vi "Plant Catalog W3.vi"() -> ()   [LabVIEW 2021, in "Tree Map.lvlib"]
doc: "<b>Author:</b> Piotr Kruczkowski <PrimaryKey>\n<b>License:</b> NewBSD\n\nCopyright (c) 2019, National Instruments\nAll rights reserved.\n\nRedistribution and use in source and binary forms, with or without\nmodification, are permitted provided that the following conditions are met:\n1. Redistributions of source code must retain the above copyright\n notice, this list of conditions and the following disclaimer.\n2. Redistributions in binary form must reproduce the above copyright\n notice, this list of conditions and the following disclaimer in the\n documentation and/or other materials provided with the distribution.\n3. Neither the name of National Instruments nor the\n names of its contributors may be used to endorse or promote products\n derived from this software without specific prior written permission.\n\nTHIS SOFTWARE IS PROVIDED BY National Instruments ''AS IS'' AND ANY\nEXPRESS OR IMPLIED WARRANTIES, INCLUDING, BUT NOT LIMITED TO, THE IMPLIED\nWARRANTIES OF MERCHANTABILITY AND FITNESS FOR A PARTICULAR PURPOSE ARE\nDISCLAIMED. IN NO EVENT SHALL National Instruments BE LIABLE FOR ANY\nDIRECT, INDIRECT, INCIDENTAL, SPECIAL, EXEMPLARY, OR CONSEQUENTIAL DAMAGES\n(INCLUDING, BUT NOT LIMITED TO, PROCUREMENT OF SUBSTITUTE GOODS OR SERVICES;\nLOSS OF USE, DATA, OR PROFITS; OR BUSINESS INTERRUPTION) HOWEVER CAUSED AND\nON ANY THEORY OF LIABILITY, WHETHER IN CONTRACT, STRICT LIABILITY, OR TORT\n(INCLUDING NEGLIGENCE OR OTHERWISE) ARISING IN ANY WAY OUT OF THE USE OF THIS\nSOFTWARE, EVEN IF ADVISED OF THE POSSIBILITY OF SUCH DAMAGE."
uses:
  <vilib>/National Instruments/Tree Map/Tree Map.lvlib
  <vilib>/National Instruments/Tree Map/API/List Roots.vi
  <vilib>/National Instruments/Tree Map/Utility/Into Tree Control Items.vi
panel:
  out "Array":string[](array[string])
  out "COMMON Unique Paths Set":set{string}(c389)={"\\CATALOG\\PLANT\\COMMON", "\\CATALOG\\PLANT_000000\\COMMON", "\\CATALOG\\PLANT_000001\\COMMON", "\\CATALOG\\PLANT_000002\\COMMON", "\\CATALOG\\PLANT_000003\\COMMON", "\\CATALOG\\PLANT_000004\\COMMON", "\\CATALOG\\PLANT_000005\\COMMON", "\\CATALOG\\PLANT_000006\\COMMON", "\\CATALOG\\PLANT_000007\\COMMON", "\\CATALOG\\PLANT_000008\\COMMON", "\\CATALOG\\PLANT_000009\\COMMON", "\\CATALOG\\PLANT_000010\\COMMON", "\\CATALOG\\PLANT_000011\\COMMON", "\\CATALOG\\PLANT_000012\\COMMON", "\\CATALOG\\PLANT_000013\\COMMON", "\\CATALOG\\PLANT_000014\\COMMON", "\\CATALOG\\PLANT_000015\\COMMON", "\\CATALOG\\PLANT_000016\\COMMON", "\\CATALOG\\PLANT_000017\\COMMON", "\\CATALOG\\PLANT_000018\\COMMON", "\\CATALOG\\PLANT_000019\\COMMON", "\\CATALOG\\PLANT_000020\\COMMON", "\\CATALOG\\PLANT_000021\\COMMON", "\\CATALOG\\PLANT_000022\\COMMON", "\\CATALOG\\PLANT_000023\\COMMON", "\\CATALOG\\PLANT_000024\\COMMON", "\\CATALOG\\PLANT_000025\\COMMON", "\\CATALOG\\PLANT_000026\\COMMON", "\\CATALOG\\PLANT_000027\\COMMON", "\\CATALOG\\PLANT_000028\\COMMON", "\\CATALOG\\PLANT_000029\\COMMON", "\\CATALOG\\PLANT_000030\\COMMON", "\\CATALOG\\PLANT_000031\\COMMON", "\\CATALOG\\PLANT_000032\\COMMON", "\\CATALOG\\PLANT_000033\\COMMON", "\\CATALOG\\PLANT_000034\\COMMON"}
  out "Botanical Data":string[](array[string])=["Sanguinaria canadensis", "Aquilegia canadensis", "Caltha palustris", "Caltha palustris", "Dicentra cucullaria", "Asarum canadense", "Hepatica americana", "Hepatica americana", "Arisaema triphyllum", "Podophyllum peltatum", "Phlox divaricata", "Phlox divaricata", "Claytonia Virginica", "Trillium grandiflorum", "Trillium grandiflorum", "Erythronium americanum", "Erythronium americanum", "Erythronium americanum", "Anemone blanda", "Anemone blanda", "Monarda didyma", "Monarda didyma", "Rudbeckia hirta", "Ranunculus", "Ranunculus", "Asclepias tuberosa", "Potentilla", "Oenothera", "Gentiana", "Gentiana", "Polemonium caeruleum", "Polemonium caeruleum", "Eschscholzia californica", "Dodecatheon", "Cimicifuga", "Lobelia cardinalis"]
  out "BOTANICAL Unique Paths Set":set{string}(c389)={"\\CATALOG\\PLANT\\BOTANICAL", "\\CATALOG\\PLANT_000000\\BOTANICAL", "\\CATALOG\\PLANT_000001\\BOTANICAL", "\\CATALOG\\PLANT_000002\\BOTANICAL", "\\CATALOG\\PLANT_000003\\BOTANICAL", "\\CATALOG\\PLANT_000004\\BOTANICAL", "\\CATALOG\\PLANT_000005\\BOTANICAL", "\\CATALOG\\PLANT_000006\\BOTANICAL", "\\CATALOG\\PLANT_000007\\BOTANICAL", "\\CATALOG\\PLANT_000008\\BOTANICAL", "\\CATALOG\\PLANT_000009\\BOTANICAL", "\\CATALOG\\PLANT_000010\\BOTANICAL", "\\CATALOG\\PLANT_000011\\BOTANICAL", "\\CATALOG\\PLANT_000012\\BOTANICAL", "\\CATALOG\\PLANT_000013\\BOTANICAL", "\\CATALOG\\PLANT_000014\\BOTANICAL", "\\CATALOG\\PLANT_000015\\BOTANICAL", "\\CATALOG\\PLANT_000016\\BOTANICAL", "\\CATALOG\\PLANT_000017\\BOTANICAL", "\\CATALOG\\PLANT_000018\\BOTANICAL", "\\CATALOG\\PLANT_000019\\BOTANICAL", "\\CATALOG\\PLANT_000020\\BOTANICAL", "\\CATALOG\\PLANT_000021\\BOTANICAL", "\\CATALOG\\PLANT_000022\\BOTANICAL", "\\CATALOG\\PLANT_000023\\BOTANICAL", "\\CATALOG\\PLANT_000024\\BOTANICAL", "\\CATALOG\\PLANT_000025\\BOTANICAL", "\\CATALOG\\PLANT_000026\\BOTANICAL", "\\CATALOG\\PLANT_000027\\BOTANICAL", "\\CATALOG\\PLANT_000028\\BOTANICAL", "\\CATALOG\\PLANT_000029\\BOTANICAL", "\\CATALOG\\PLANT_000030\\BOTANICAL", "\\CATALOG\\PLANT_000031\\BOTANICAL", "\\CATALOG\\PLANT_000032\\BOTANICAL", "\\CATALOG\\PLANT_000033\\BOTANICAL", "\\CATALOG\\PLANT_000034\\BOTANICAL"}
  in  "Tree Control":string(tree)
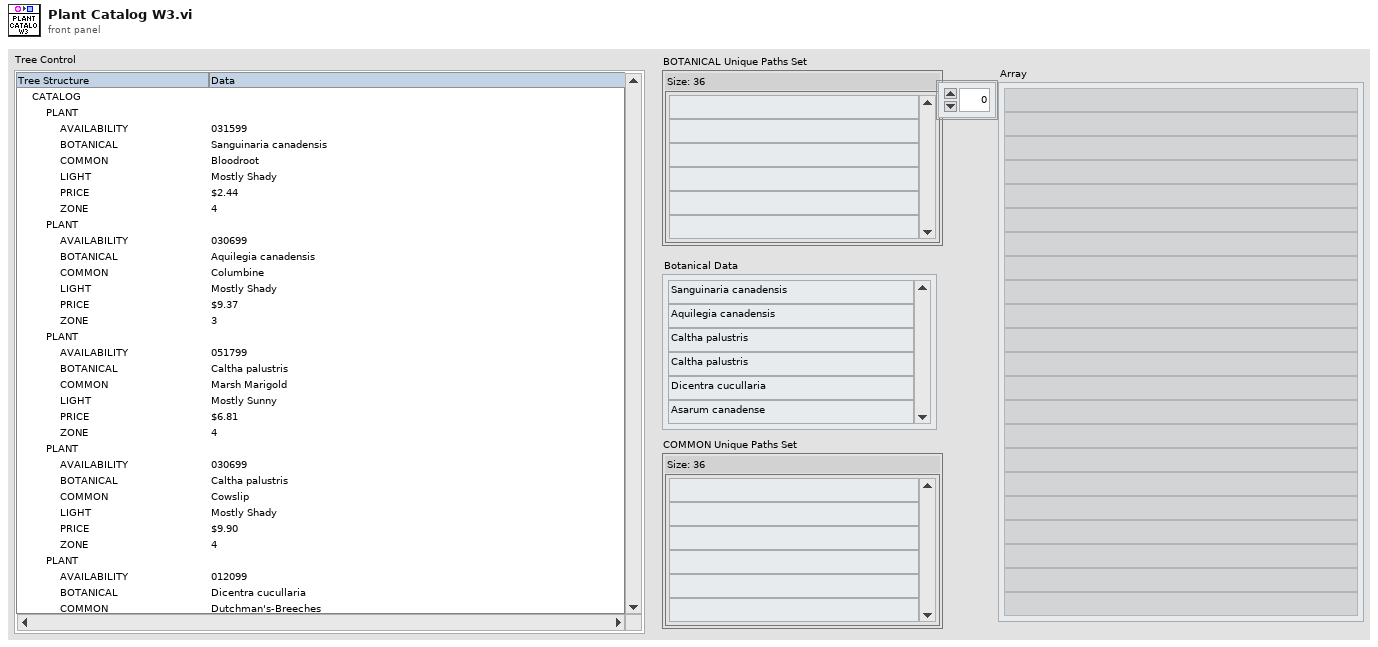
[diagram p1: front panel]
types:
  T1 = typedef "Tree Map.lvlib/Tree Map Data.ctl" = map{string, cluster{"Child Paths Set":set{string}, "Name":string, "Data":string, "Attributes":map{string, string}}}
  T2 = cluster{"Left Cell String":string, "Child Text":string[], "Child Tag":string, "Item Indent":i32, "Child Only?":bool, "Glyph Index":i32}[]
  T3 = cluster{"Child Paths Set":set{string}, "Name":string, "Data":string, "Attributes":map{string, string}}
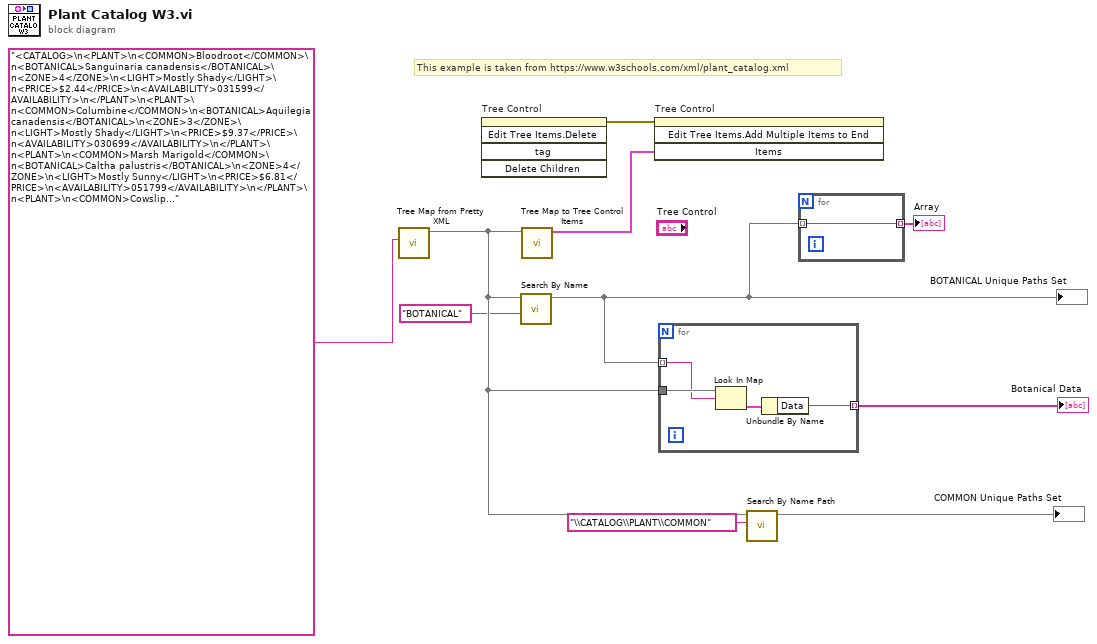
[diagram p0: block diagram]
diagram:
  # "This example is taken from https://www.w3schools.com/xml/plant_catalog.xml"
  n1 = call <vilib>:"Tree Map from Pretty XML.vi"("Pretty XML"="<CATALOG>\n<PLANT>\n<COMMON>Bloodroot</COMMON>\n<BOTANICAL>Sanguinaria canadensis</BOTANICAL>\n<ZONE>4</ZONE>\n<LIGHT>Mostly Shady</LIGHT>\n<PRICE>$2.44</PRICE>\n<AVAILABILITY>031599</AVAILABILITY>\n</PLANT>\n<PLANT>\n<COMMON>Columbine</COMMON>\n<BOTANICAL>Aquilegia canadensis</BOTANICAL>\n<ZONE>3</ZONE>\n<LIGHT>Mostly Shady</LIGHT>\n<PRICE>$9.37</PRICE>\n<AVAILABILITY>030699</AVAILABILITY>\n</PLANT>\n<PLANT>\n<COMMON>Marsh Marigold</COMMON>\n<BOTANICAL>Caltha palustris</BOTANICAL>\n<ZONE>4</ZONE>\n<LIGHT>Mostly Sunny</LIGHT>\n<PRICE>$6.81</PRICE>\n<AVAILABILITY>051799</AVAILABILITY>\n</PLANT>\n<PLANT>\n<COMMON>Cowslip</COMMON>\n<BOTANICAL>Caltha palustris</BOTANICAL>\n<ZONE>4</ZONE>\n<LIGHT>Mostly Shady</LIGHT>\n<PRICE>$9.90</PRICE>\n<AVAILABILITY>030699</AVAILABILITY>\n</PLANT>\n<PLANT>\n<COMMON>Dutchman's-Breeches</COMMON>\n<BOTANICAL>Dicentra cucullaria</BOTANICAL>\n<ZONE>3</ZONE>\n<LIGHT>Mostly Shady</LIGHT>\n<PRICE>$6.44</PRICE>\n<AVAILABILITY>012099</AVAILABILITY>\n</PLANT>\n<PLANT>\n<COMMON>Ginger, Wild</COMMON>\n<BOTANICAL>Asarum canadense</BOTANICAL>\n<ZONE>3</ZONE>\n<LIGHT>Mostly Shady</LIGHT>\n<PRICE>$9.03</PRICE>\n<AVAILABILITY>041899</AVAILABILITY>\n</PLANT>\n<PLANT>\n<COMMON>Hepatica</COMMON>\n<BOTANICAL>Hepatica americana</BOTANICAL>\n<ZONE>4</ZONE>\n<LIGHT>Mostly Shady</LIGHT>\n<PRICE>$4.45</PRICE>\n<AVAILABILITY>012699</AVAILABILITY>\n</PLANT>\n<PLANT>\n<COMMON>Liverleaf</COMMON>\n<BOTANICAL>Hepatica americana</BOTANICAL>\n<ZONE>4</ZONE>\n<LIGHT>Mostly Shady</LIGHT>\n<PRICE>$3.99</PRICE>\n<AVAILABILITY>010299</AVAILABILITY>\n</PLANT>\n<PLANT>\n<COMMON>Jack-In-The-Pulpit</COMMON>\n<BOTANICAL>Arisaema triphyllum</BOTANICAL>\n<ZONE>4</ZONE>\n<LIGHT>Mostly Shady</LIGHT>\n<PRICE>$3.23</PRICE>\n<AVAILABILITY>020199</AVAILABILITY>\n</PLANT>\n<PLANT>\n<COMMON>Mayapple</COMMON>\n<BOTANICAL>Podophyllum peltatum</BOTANICAL>\n<ZONE>3</ZONE>\n<LIGHT>Mostly Shady</LIGHT>\n<PRICE>$2.98</PRICE>\n<AVAILABILITY>060599</AVAILABILITY>\n</PLANT>\n<PLANT>\n<COMMON>Phlox, Woodland</COMMON>\n<BOTANICAL>Phlox divaricata</BOTANICAL>\n<ZONE>3</ZONE>\n<LIGHT>Sun or Shade</LIGHT>\n<PRICE>$2.80</PRICE>\n<AVAILABILITY>012299</AVAILABILITY>\n</PLANT>\n<PLANT>\n<COMMON>Phlox, Blue</COMMON>\n<BOTANICAL>Phlox divaricata</BOTANICAL>\n<ZONE>3</ZONE>\n<LIGHT>Sun or Shade</LIGHT>\n<PRICE>$5.59</PRICE>\n<AVAILABILITY>021699</AVAILABILITY>\n</PLANT>\n<PLANT>\n<COMMON>Spring-Beauty</COMMON>\n<BOTANICAL>Claytonia Virginica</BOTANICAL>\n<ZONE>7</ZONE>\n<LIGHT>Mostly Shady</LIGHT>\n<PRICE>$6.59</PRICE>\n<AVAILABILITY>020199</AVAILABILITY>\n</PLANT>\n<PLANT>\n<COMMON>Trillium</COMMON>\n<BOTANICAL>Trillium grandiflorum</BOTANICAL>\n<ZONE>5</ZONE>\n<LIGHT>Sun or Shade</LIGHT>\n<PRICE>$3.90</PRICE>\n<AVAILABILITY>042999</AVAILABILITY>\n</PLANT>\n<PLANT>\n<COMMON>Wake Robin</COMMON>\n<BOTANICAL>Trillium grandiflorum</BOTANICAL>\n<ZONE>5</ZONE>\n<LIGHT>Sun or Shade</LIGHT>\n<PRICE>$3.20</PRICE>\n<AVAILABILITY>022199</AVAILABILITY>\n</PLANT>\n<PLANT>\n<COMMON>Violet, Dog-Tooth</COMMON>\n<BOTANICAL>Erythronium americanum</BOTANICAL>\n<ZONE>4</ZONE>\n<LIGHT>Shade</LIGHT>\n<PRICE>$9.04</PRICE>\n<AVAILABILITY>020199</AVAILABILITY>\n</PLANT>\n<PLANT>\n<COMMON>Trout Lily</COMMON>\n<BOTANICAL>Erythronium americanum</BOTANICAL>\n<ZONE>4</ZONE>\n<LIGHT>Shade</LIGHT>\n<PRICE>$6.94</PRICE>\n<AVAILABILITY>032499</AVAILABILITY>\n</PLANT>\n<PLANT>\n<COMMON>Adder's-Tongue</COMMON>\n<BOTANICAL>Erythronium americanum</BOTANICAL>\n<ZONE>4</ZONE>\n<LIGHT>Shade</LIGHT>\n<PRICE>$9.58</PRICE>\n<AVAILABILITY>041399</AVAILABILITY>\n</PLANT>\n<PLANT>\n<COMMON>Anemone</COMMON>\n<BOTANICAL>Anemone blanda</BOTANICAL>\n<ZONE>6</ZONE>\n<LIGHT>Mostly Shady</LIGHT>\n<PRICE>$8.86</PRICE>\n<AVAILABILITY>122698</AVAILABILITY>\n</PLANT>\n<PLANT>\n<COMMON>Grecian Windflower</COMMON>\n<BOTANICAL>Anemone blanda</BOTANICAL>\n<ZONE>6</ZONE>\n<LIGHT>Mostly Shady</LIGHT>\n<PRICE>$9.16</PRICE>\n<AVAILABILITY>071099</AVAILABILITY>\n</PLANT>\n<PLANT>\n<COMMON>Bee Balm</COMMON>\n<BOTANICAL>Monarda didyma</BOTANICAL>\n<ZONE>4</ZONE>\n<LIGHT>Shade</LIGHT>\n<PRICE>$4.59</PRICE>\n<AVAILABILITY>050399</AVAILABILITY>\n</PLANT>\n<PLANT>\n<COMMON>Bergamot</COMMON>\n<BOTANICAL>Monarda didyma</BOTANICAL>\n<ZONE>4</ZONE>\n<LIGHT>Shade</LIGHT>\n<PRICE>$7.16</PRICE>\n<AVAILABILITY>042799</AVAILABILITY>\n</PLANT>\n<PLANT>\n<COMMON>Black-Eyed Susan</COMMON>\n<BOTANICAL>Rudbeckia hirta</BOTANICAL>\n<ZONE>Annual</ZONE>\n<LIGHT>Sunny</LIGHT>\n<PRICE>$9.80</PRICE>\n<AVAILABILITY>061899</AVAILABILITY>\n</PLANT>\n<PLANT>\n<COMMON>Buttercup</COMMON>\n<BOTANICAL>Ranunculus</BOTANICAL>\n<ZONE>4</ZONE>\n<LIGHT>Shade</LIGHT>\n<PRICE>$2.57</PRICE>\n<AVAILABILITY>061099</AVAILABILITY>\n</PLANT>\n<PLANT>\n<COMMON>Crowfoot</COMMON>\n<BOTANICAL>Ranunculus</BOTANICAL>\n<ZONE>4</ZONE>\n<LIGHT>Shade</LIGHT>\n<PRICE>$9.34</PRICE>\n<AVAILABILITY>040399</AVAILABILITY>\n</PLANT>\n<PLANT>\n<COMMON>Butterfly Weed</COMMON>\n<BOTANICAL>Asclepias tuberosa</BOTANICAL>\n<ZONE>Annual</ZONE>\n<LIGHT>Sunny</LIGHT>\n<PRICE>$2.78</PRICE>\n<AVAILABILITY>063099</AVAILABILITY>\n</PLANT>\n<PLANT>\n<COMMON>Cinquefoil</COMMON>\n<BOTANICAL>Potentilla</BOTANICAL>\n<ZONE>Annual</ZONE>\n<LIGHT>Shade</LIGHT>\n<PRICE>$7.06</PRICE>\n<AVAILABILITY>052599</AVAILABILITY>\n</PLANT>\n<PLANT>\n<COMMON>Primrose</COMMON>\n<BOTANICAL>Oenothera</BOTANICAL>\n<ZONE>3 - 5</ZONE>\n<LIGHT>Sunny</LIGHT>\n<PRICE>$6.56</PRICE>\n<AVAILABILITY>013099</AVAILABILITY>\n</PLANT>\n<PLANT>\n<COMMON>Gentian</COMMON>\n<BOTANICAL>Gentiana</BOTANICAL>\n<ZONE>4</ZONE>\n<LIGHT>Sun or Shade</LIGHT>\n<PRICE>$7.81</PRICE>\n<AVAILABILITY>051899</AVAILABILITY>\n</PLANT>\n<PLANT>\n<COMMON>Blue Gentian</COMMON>\n<BOTANICAL>Gentiana</BOTANICAL>\n<ZONE>4</ZONE>\n<LIGHT>Sun or Shade</LIGHT>\n<PRICE>$8.56</PRICE>\n<AVAILABILITY>050299</AVAILABILITY>\n</PLANT>\n<PLANT>\n<COMMON>Jacob's Ladder</COMMON>\n<BOTANICAL>Polemonium caeruleum</BOTANICAL>\n<ZONE>Annual</ZONE>\n<LIGHT>Shade</LIGHT>\n<PRICE>$9.26</PRICE>\n<AVAILABILITY>022199</AVAILABILITY>\n</PLANT>\n<PLANT>\n<COMMON>Greek Valerian</COMMON>\n<BOTANICAL>Polemonium caeruleum</BOTANICAL>\n<ZONE>Annual</ZONE>\n<LIGHT>Shade</LIGHT>\n<PRICE>$4.36</PRICE>\n<AVAILABILITY>071499</AVAILABILITY>\n</PLANT>\n<PLANT>\n<COMMON>California Poppy</COMMON>\n<BOTANICAL>Eschscholzia californica</BOTANICAL>\n<ZONE>Annual</ZONE>\n<LIGHT>Sun</LIGHT>\n<PRICE>$7.89</PRICE>\n<AVAILABILITY>032799</AVAILABILITY>\n</PLANT>\n<PLANT>\n<COMMON>Shooting Star</COMMON>\n<BOTANICAL>Dodecatheon</BOTANICAL>\n<ZONE>Annual</ZONE>\n<LIGHT>Mostly Shady</LIGHT>\n<PRICE>$8.60</PRICE>\n<AVAILABILITY>051399</AVAILABILITY>\n</PLANT>\n<PLANT>\n<COMMON>Snakeroot</COMMON>\n<BOTANICAL>Cimicifuga</BOTANICAL>\n<ZONE>Annual</ZONE>\n<LIGHT>Shade</LIGHT>\n<PRICE>$5.63</PRICE>\n<AVAILABILITY>071199</AVAILABILITY>\n</PLANT>\n<PLANT>\n<COMMON>Cardinal Flower</COMMON>\n<BOTANICAL>Lobelia cardinalis</BOTANICAL>\n<ZONE>2</ZONE>\n<LIGHT>Shade</LIGHT>\n<PRICE>$3.02</PRICE>\n<AVAILABILITY>022299</AVAILABILITY>\n</PLANT>\n</CATALOG>") -> ("Tree Map Out"=w7:T1)  [unwired: 9 in, 1 out]
  n2 = invoke on="Tree Control" class="Tree (strict)" method="Edit Tree Items.Delete"() -> (error out=w10:errorcluster)  [unwired: 5 in, 4 out]
  n3 = call <vilib>:"Search By Name.vi"("Node Name"="BOTANICAL" ("Path or Node Name"), "Tree Map In"=w7) -> ("Unique Paths Set"=w2:set{string})  [unwired: 9 in]
  "BOTANICAL Unique Paths Set" <- w2
  n4 = call <vilib>:"Tree Map to Tree Control Items.vi"("Tree Map In"=w7) -> ("Tree Control Items"=w9:T2)  [unwired: 10 in]
  n5 = invoke on="Tree Control" class="Tree (strict)" method="Edit Tree Items.Add Multiple Items to End"(error in=w10, "Items"=w9) -> ()  [unwired: 2 in, 4 out]
  n6 = for {
    tunnel: w2 -> [w13] mode=indexing
    tunnel: w7 -> [w14]
    tunnel: [w11] -> w8 mode=indexing
    n7 = Look In Map(map=w14, key=w13) -> (value=w12:T3)  [unwired: 1 in, 1 out]
    n8 = Unbundle By Name(w12) -> ("Data"=w11:string)
  }
  "Botanical Data" <- w8
  n9 = call <vilib>:"Search By Name Path.vi"("Node Name Path"="\\CATALOG\\PLANT\\COMMON" ("Special Name Path"), "Tree Map In"=w7) -> ("Unique Paths Set"=→"COMMON Unique Paths Set":set{string})  [unwired: 9 in]
  n10 = for {
    tunnel: w2 -> [w15] mode=indexing
    tunnel: [w15] -> w1 mode=indexing
  }
  "Array" <- w1
